vi "Stop and Clear Processes.vi"(6 "This VI":refnum<vi>, 8 "error in (no error)":errorcluster, 11 "VI Refs In":refnum<vi>[](array[refnum])) -> (0 "error out":errorcluster)   [LabVIEW 2013, in "J1939 Addon Engine.lvlib"]
uses:
  J1939 Addon Engine.lvlib
  Inline Async API/Inline Async API.lvlib
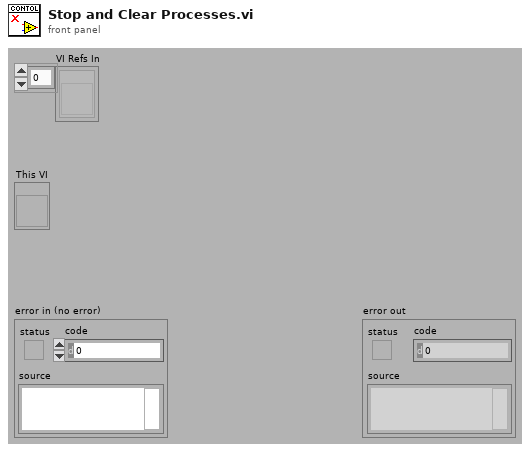
[diagram p1: front panel]
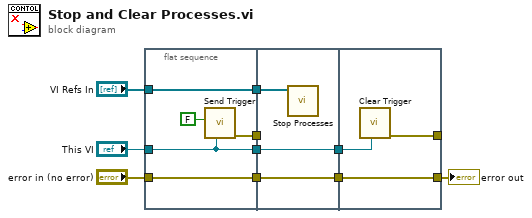
[diagram p0: block diagram]
diagram:
  n1 = flat-sequence {
    tunnel: "error in (no error)" -> [w12]
    tunnel: "This VI" -> [w14]
    tunnel: [w15] -> w7
    tunnel: "VI Refs In" -> [w15]
    tunnel: [w14] -> w4
    tunnel: [w13] -> w3
    tunnel: [w12] -> w1
    tunnel: w7 -> [w18]
    tunnel: [w17] -> w5
    tunnel: w4 -> [w17]
    tunnel: w3 -> [_]
    tunnel: [w16] -> w2
    tunnel: w1 -> [w16]
    tunnel: [w19] -> w10
    tunnel: w5 -> [w21]
    tunnel: [w20] -> _
    tunnel: w2 -> [w19]
    frame #0 {
      n2 = call "Send Trigger.vi"("Parent VI"=w14, "notification"=FALSE) -> ("error out"=w13:errorcluster)  [unwired: 9 in]
    }
    frame #1 {
      n3 = call "Stop Processes.vi"("VI Refs"=w18) -> ()  [unwired: 11 in]
    }
    frame #2 {
      n4 = call "Clear Trigger.vi"("Parent VI"=w21) -> ("error out"=w20:errorcluster)  [unwired: 10 in]
    }
  }
  "error out" <- w10
